vi "Scripting_GetNodeInfo.vi"(1 "Node Refnum Or Constrol/Indicator/Constant":refnum<vi>, 5 "error in (no error)":errorcluster) -> (14 "OK":bool, 15 "NodeInfo":T1, 19 "error out":errorcluster)   [LabVIEW 2012]
uses:
  <resource>/Framework/Providers/Open_GDS/ClassProviders/Common/ScriptingFunctions/Scripting_NodeInfo.ctl
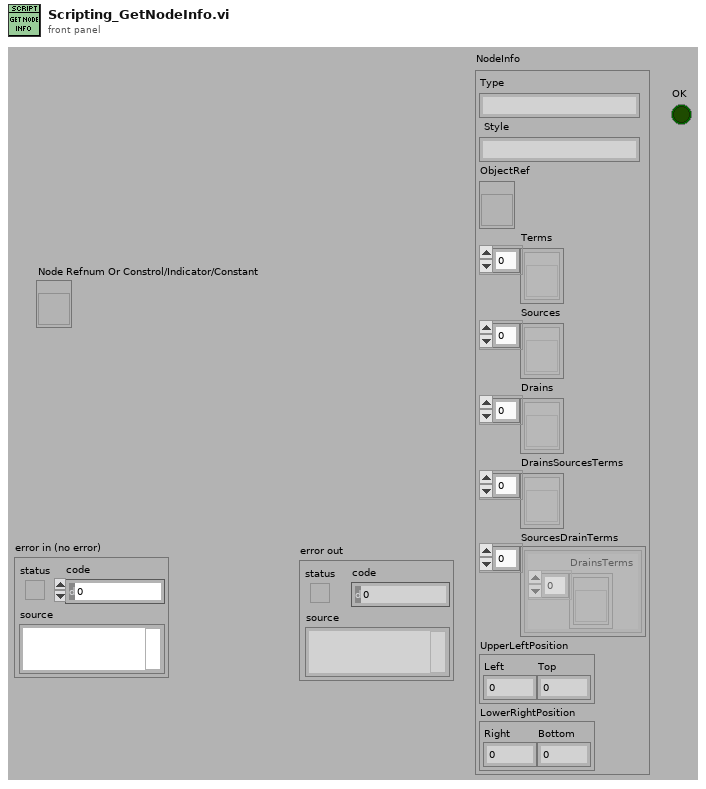
[diagram p1: front panel]
types:
  T1 = typedef "Scripting_NodeInfo.ctl" = cluster{"Type":string, "Style":string, "ObjectRef":refnum<vi>, "Terms":refnum<vi>[], "Sources":refnum<vi>[], "Drains":refnum<vi>[], "DrainsSourcesTerms":refnum<vi>[], "SourcesDrainTerms":cluster{"DrainsTerms":refnum<vi>[]}[], "UpperLeftPosition":cluster{"Left":i32, "Top":i32}, "LowerRightPosition":cluster{"Right":i32, "Bottom":i32}}
  T2 = typedef "LVPositionTypeDef.ctl" = cluster{"Left":i32, "Top":i32}
  T3 = typedef "LVBoundsTypeDef.ctl" = cluster{"Width":u32, "Height":u32}
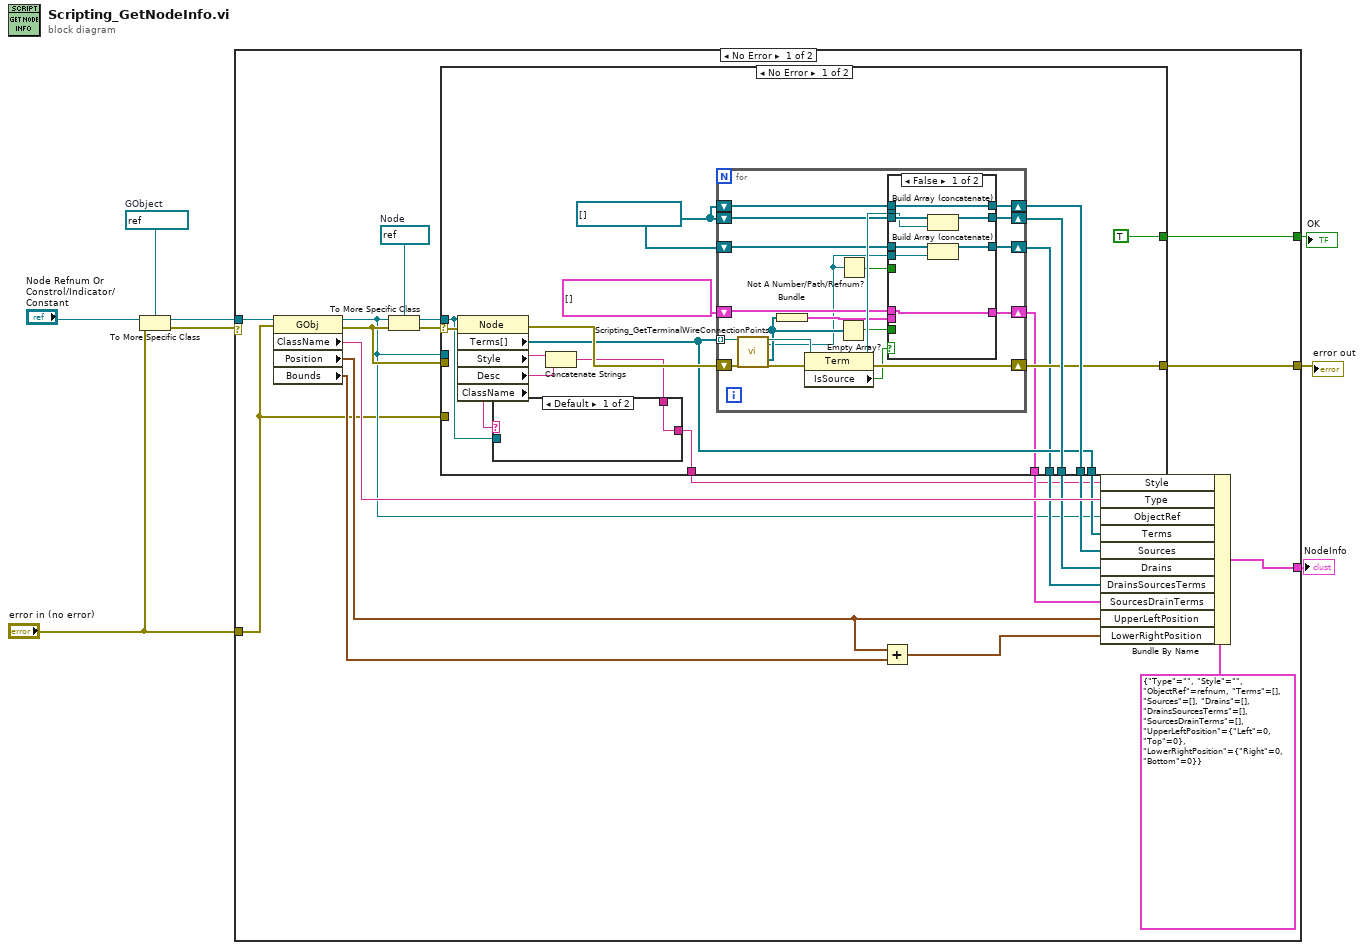
[diagram p0: block diagram]
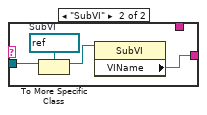
[diagram p2: hidden frame]
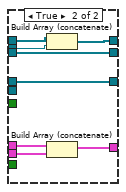
[diagram p3: hidden frame]
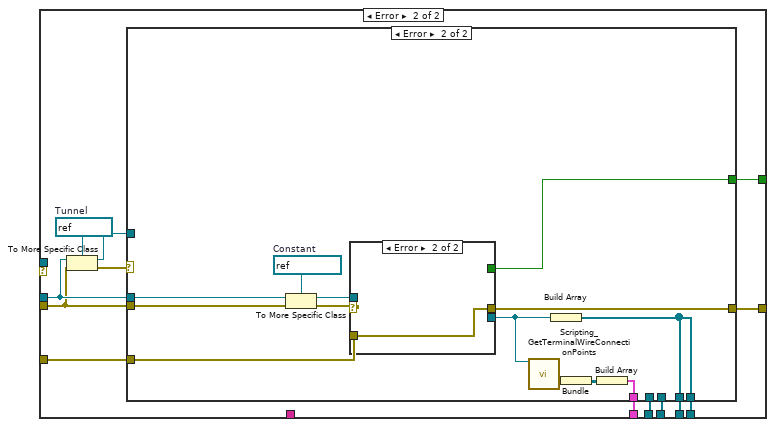
[diagram p4: hidden frame]
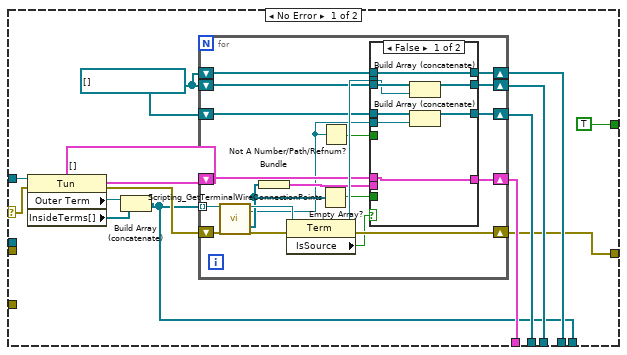
[diagram p5: hidden frame]
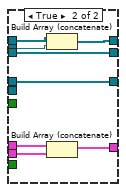
[diagram p6: hidden frame]
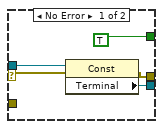
[diagram p7: hidden frame]
diagram:
  w3 = refnum<vi> refnum  # GObject
  n1 = To More Specific Class(target class=w3, reference="Node Refnum Or Constrol/Indicator/Constant", error in="error in (no error)") -> (specific class reference=w2:refnum<vi>, error out=w1:errorcluster)
  n2 = case shown="No Error" w1 {
    tunnel: [w23 w170] -> w8
    tunnel: [w22 _] -> w7
    tunnel: [w14 _] -> w6
    tunnel: "error in (no error)" -> [w9 w170]
    tunnel: w2 -> [w11 _]
    frame No Error {
      w17 = refnum<vi> refnum  # Node
      n3 = property class="GObj"(reference=w11, error in=w9) -> (reference out=w12:refnum<vi>, error out=w13:errorcluster, "ClassName"=w28:string, "Position"=w21:T2, "Bounds"=w20:T3)
      n4 = To More Specific Class(target class=w17, reference=w12, error in=w13) -> (specific class reference=w15:refnum<vi>, error out=w16:errorcluster)
      n5 = case shown="No Error" w16 {
        selector: w16 -> [w41 _]
        tunnel: [w46 w100] -> w27
        tunnel: [w45 w89] -> w26
        tunnel: [w36 w90] -> w25
        tunnel: [w38 w99] -> w24
        tunnel: [w44 w98] -> w23
        tunnel: [w42 w88] -> w18
        tunnel: w15 -> [w33 _]
        tunnel: w12 -> [_ w95]
        tunnel: [TRUE w96] -> w14
        tunnel: w13 -> [_ w91]
        tunnel: [w34 _] -> w10
        tunnel: w9 -> [_ w97]
        frame No Error {
          w37 = refnum<vi>[] []
          n6 = property class="Node"(reference=w33, error in=w41) -> (error out=w43:errorcluster, "Terms[]"=w42:refnum<vi>[], "Style"=w32:string, "Desc"=w31:string, "ClassName"=w35:string)  [unwired: 1 out]
          n7 = Concatenate Strings(w32, w31) -> (w30:string)
          n8 = case shown="Default" w35 {
            tunnel: w30 -> [w47 _]
            tunnel: [w47 w48] -> w34
            tunnel: w33 -> [_ w51]
            frame Default {
            }
            frame "SubVI" {
              w50 = refnum<vi> refnum  # SubVI
              n9 = To More Specific Class(target class=w50, reference=w51) -> (specific class reference=w49:refnum<vi>)  [unwired: 1 in, 1 out]
              n10 = property class="SubVI"(reference=w49) -> ("VIName"=w48:string)  [unwired: 1 in, 2 out]
            }
          }
          n11 = for {
            tunnel: w42 -> [w71] mode=indexing
            shift-right: [w68] -> w44
            shift-left: w43 -> [w70]
            shift-right: [w65] -> w46
            shift-left: w37 -> [w64]
            shift-right: [w61] -> w45
            shift-left: w37 -> [w62]
            shift-right: [w60] -> w38
            shift-left: cluster{"AllWireTerminalDrains":refnum<vi>[]}[] [] -> [w59]
            shift-right: [w57] -> w36
            shift-left: w37 -> [w56]
            n12 = call <resource>:"Scripting_GetTerminalWireConnectionPoints.vi"("Term Refnum In"=w71, "error in"=w70) -> ("Term Refnum Out"=w67:refnum<vi>, "WireTermSource"=w53:refnum<vi>, "AllWireTerminalDrains"=w55:refnum<vi>[], "error out"=w69:errorcluster)  [unwired: 9 in, 5 out]
            n13 = Bundle("AllWireTerminalDrains"=w55) -> (w58:cluster{"AllWireTerminalDrains":refnum<vi>[]})  [unwired: 1 in]
            n14 = property class="Term"(reference=w67, error in=w69) -> (reference out=w63:refnum<vi>, error out=w68:errorcluster, "IsSource"=w66:bool)
            n15 = Empty Array?(array=w55) -> (empty?=w54:bool)
            n16 = Not A Number/Path/Refnum?(number/path/refnum=w53) -> (NaN/Path/Refnum?=w52:bool)
            n17 = case shown="False" w66 {
              tunnel: [w79 w87] -> w65
              tunnel: w64 -> [w79 w86]
              tunnel: w63 -> [w76 w85]
              tunnel: [w77 w84] -> w61
              tunnel: w62 -> [w78 w84]
              tunnel: [w75 w83] -> w60
              tunnel: w59 -> [w75 w82]
              tunnel: w58 -> [_ w81]
              tunnel: [w74 w80] -> w57
              tunnel: w56 -> [w73 w80]
              tunnel: w53 -> [w72 _]
              tunnel: w54 -> [_ _]
              tunnel: w52 -> [_ _]
              frame False {
                n18 = Build Array (concatenate)(w78, w76) -> (w77:refnum<vi>[])
                n19 = Build Array (concatenate)(w73, w72) -> (w74:refnum<vi>[])
              }
              frame True {
                n20 = Build Array (concatenate)(w86, w85) -> (w87:refnum<vi>[])
                n21 = Build Array (concatenate)(w82, w81) -> (w83:cluster{"AllWireTerminalDrains":refnum<vi>[]}[])
              }
            }
          }
        }
        frame Error {
          w94 = refnum<vi> refnum  # Tunnel
          n22 = To More Specific Class(target class=w94, reference=w95, error in=w91) -> (specific class reference=w92:refnum<vi>, error out=w93:errorcluster)
          n23 = case shown="Error" w93 {
            selector: w93 -> [w103 _]
            tunnel: w91 -> [_ w162]
            tunnel: [w106 w151] -> w100
            tunnel: [w109 w156] -> w99
            tunnel: [w105 w155] -> w98
            tunnel: w97 -> [_ w154]
            tunnel: [TRUE w153] -> w96
            tunnel: w95 -> [_ w152]
            tunnel: w92 -> [w114 _]
            tunnel: [w108 _] -> w90
            tunnel: [w107 _] -> w89
            tunnel: [w102 w151] -> w88
            frame No Error {
              w110 = refnum<vi>[] []
              n24 = property class="Tun"(reference=w114, error in=w103) -> (error out=w104:errorcluster, "Outer Term"=w113:refnum<vi>, "InsideTerms[]"=w112:refnum<vi>[])  [unwired: 1 out]
              n25 = Build Array (concatenate)(w113, w112) -> (w102:refnum<vi>[])
              n26 = for {
                tunnel: w102 -> [w134] mode=indexing
                shift-right: [w131] -> w105
                shift-left: w104 -> [w133]
                shift-right: [w128] -> w106
                shift-left: w110 -> [w127]
                shift-right: [w124] -> w107
                shift-left: w110 -> [w125]
                shift-right: [w123] -> w109
                shift-left: cluster{"AllWireTerminalDrains":refnum<vi>[]}[] [] -> [w122]
                shift-right: [w120] -> w108
                shift-left: w110 -> [w119]
                n27 = call <resource>:"Scripting_GetTerminalWireConnectionPoints.vi"("Term Refnum In"=w134, "error in"=w133) -> ("Term Refnum Out"=w130:refnum<vi>, "WireTermSource"=w116:refnum<vi>, "AllWireTerminalDrains"=w118:refnum<vi>[], "error out"=w132:errorcluster)  [unwired: 9 in, 5 out]
                n28 = Bundle("AllWireTerminalDrains"=w118) -> (w121:cluster{"AllWireTerminalDrains":refnum<vi>[]})  [unwired: 1 in]
                n29 = property class="Term"(reference=w130, error in=w132) -> (reference out=w126:refnum<vi>, error out=w131:errorcluster, "IsSource"=w129:bool)
                n30 = Empty Array?(array=w118) -> (empty?=w117:bool)
                n31 = Not A Number/Path/Refnum?(number/path/refnum=w116) -> (NaN/Path/Refnum?=w115:bool)
                n32 = case shown="False" w129 {
                  tunnel: [w142 w150] -> w128
                  tunnel: w127 -> [w142 w149]
                  tunnel: w126 -> [w139 w148]
                  tunnel: [w140 w147] -> w124
                  tunnel: w125 -> [w141 w147]
                  tunnel: [w138 w146] -> w123
                  tunnel: w122 -> [w138 w145]
                  tunnel: w121 -> [_ w144]
                  tunnel: [w137 w143] -> w120
                  tunnel: w119 -> [w136 w143]
                  tunnel: w116 -> [w135 _]
                  tunnel: w117 -> [_ _]
                  tunnel: w115 -> [_ _]
                  frame False {
                    n33 = Build Array (concatenate)(w141, w139) -> (w140:refnum<vi>[])
                    n34 = Build Array (concatenate)(w136, w135) -> (w137:refnum<vi>[])
                  }
                  frame True {
                    n35 = Build Array (concatenate)(w149, w148) -> (w150:refnum<vi>[])
                    n36 = Build Array (concatenate)(w145, w144) -> (w146:cluster{"AllWireTerminalDrains":refnum<vi>[]}[])
                  }
                }
              }
            }
            frame Error {
              w163 = refnum<vi> refnum  # Constant
              n37 = To More Specific Class(target class=w163, reference=w152, error in=w162) -> (specific class reference=w160:refnum<vi>, error out=w161:errorcluster)
              n38 = case shown="Error" w161 {
                selector: w161 -> [w166 _]
                tunnel: w160 -> [w168 _]
                tunnel: [w167 _] -> w159
                tunnel: [w165 w169] -> w155
                tunnel: [TRUE _] -> w153
                tunnel: w154 -> [_ w169]
                frame No Error {
                  n39 = property class="Const"(reference=w168, error in=w166) -> (error out=w165:errorcluster, "Terminal"=w167:refnum<vi>)  [unwired: 1 out]
                }
                frame Error {
                }
              }
              n40 = call <resource>:"Scripting_GetTerminalWireConnectionPoints.vi"("Term Refnum In"=w159) -> ("AllWireTerminalDrains"=w158:refnum<vi>[])  [unwired: 10 in, 8 out]
              n41 = Build Array(w159) -> (w151:refnum<vi>[])
              n42 = Bundle("AllWireTerminalDrains"=w158) -> (w157:cluster{"AllWireTerminalDrains":refnum<vi>[]})  [unwired: 1 in]
              n43 = Build Array(w157) -> (w156:cluster{"AllWireTerminalDrains":refnum<vi>[]}[])
            }
          }
        }
      }
      n44 = Add(x=w21, y=w20) -> (x+y=w19:T3)
      n45 = Bundle By Name(cluster=T1 {"Type"="", "Style"="", "ObjectRef"=refnum, "Terms"=[], "Sources"=[], "Drains"=[], "DrainsSourcesTerms"=[], "SourcesDrainTerms"=[], "UpperLeftPosition"={"Left"=0, "Top"=0}, "LowerRightPosition"={"Right"=0, "Bottom"=0}} ("NodeInfo"), "Style"=w10, "Type"=w28, "ObjectRef"=w12, "Terms"=w18, "Sources"=w27, "Drains"=w26, "DrainsSourcesTerms"=w25, "SourcesDrainTerms"=w24, "UpperLeftPosition"=w21, "LowerRightPosition"=w19) -> (w22:T1)
    }
    frame Error {
    }
  }
  "error out" <- w8
  "NodeInfo" <- w7
  "OK" <- w6
